vi "HGF_Base.appendData2Variant.vi"(0 "initData":variant, 5 "error in (no error)":errorcluster) -> (14 "dup initData":variant, 19 "error out":errorcluster)   [LabVIEW 2014, in "HGF_BaseClasses.lvlib" / "HGF_Base.lvclass"]
uses:
  HGF_Base.lvclass
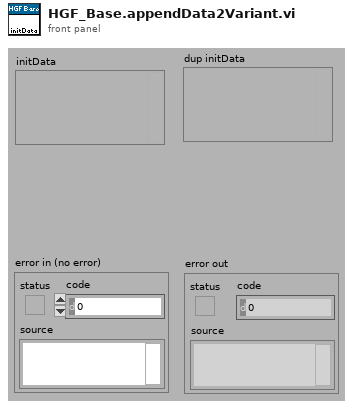
[diagram p1: front panel]
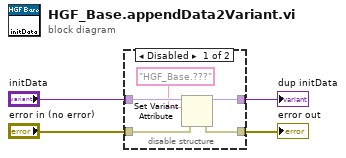
[diagram p0: block diagram]
diagram:
  n1 = disable-structure shown="Disabled" {
    disable-tunnel: "initData" -> [w9 w11]
    disable-tunnel: [w8 w11] -> w3
    disable-tunnel: "error in (no error)" -> [w7 w10]
    disable-tunnel: [w6 w10] -> w1
    frame Disabled {
      n2 = Set Variant Attribute(Variant=w9, name="HGF_Base.???", error in=w7) -> (Variant out=w8:variant, error out=w6:errorcluster)  [unwired: 1 in, 1 out]
    }
    frame Enabled {
    }
  }
  "dup initData" <- w3
  "error out" <- w1
